vi "Main - On Load.vi"(8 "error in (no error)":errorcluster, 11 "Device Item Ref in":T1 format="%.0x") -> (0 "error out":errorcluster, 3 "Device Item Ref out":T1 format="%.0x")   [LabVIEW 2026, in "SEECD System Explorer.lvlib"]
uses:
  SEECD System Explorer.lvlib
  <vilib>/NI VeriStand/Custom Device API/Custom Device API.lvlib
  <vilib>/NI VeriStand/Custom Device API/Custom Device Channel Type.ctl
  <vilib>/NI VeriStand/Custom Device API/Custom Device Channel.ctl
  <vilib>/NI VeriStand/Custom Device Tools/Custom Device Utility Library/Custom Device Utility Library.lvlib
  Shared/Globals/Scan Engine GUIDs.vi
  Shared/SEECD Shared.lvlib
  Shared/Globals/Property Strings.vi
  <vilib>/NI VeriStand/Custom Device Tools/Custom Device Utility Library/NI VeriStand - Search for All Items by GUID.vi
  Shared/Globals/String Constants.vi
  <vilib>/NI VeriStand/Custom Device API/Set Item Property (Boolean).vi
  <vilib>/NI VeriStand/Custom Device API/Get Item Property (U32).vi
  <vilib>/NI VeriStand/Custom Device API/Set Item Property (String).vi
  C:/Users/Administrator/Desktop/Jatin/All DNC DLLs/NationalInstruments.VeriStand.SystemDefinitionAPI.dll
  Jatin/All DNC DLLs/NationalInstruments.VeriStand.SystemDefinitionAPI.dll
  <vilib>/NI VeriStand/Custom Device API/Custom Device Item Ref.ctl
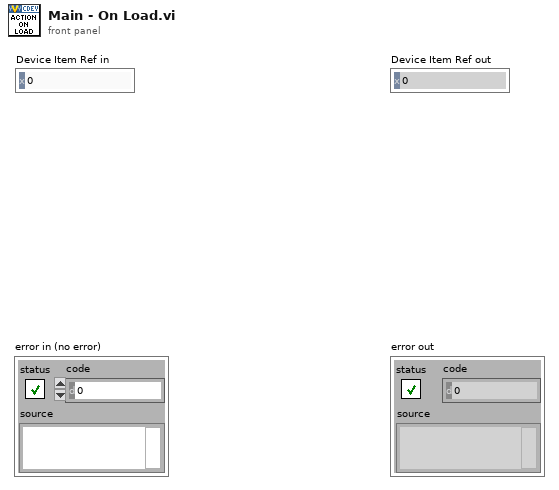
[diagram p1: front panel]
types:
  T1 = typedef "Custom Device API.lvlib/Custom Device Item Ref.ctl" = u64
  T2 = typedef "Custom Device API.lvlib/Custom Device Channel.ctl" = cluster{"Type":T3, "Units":string, "Default Value":dbl, "Faultable":bool, "Scalable":bool}
  T3 = typedef "Custom Device API.lvlib/Custom Device Channel Type.ctl" = enum16{"Input", "Output"}
  T4 = cluster{"Property Name Format String":string, "Offset":i32}
  T5 = typedef "Modules.lvlibp/Custom Device API.lvlib/Custom Device Item Ref.ctl" = u64
  T6 = typedef "Modules.lvlibp/RSI Module.lvclass/Module Models.ctl" = enum16{"Empty", "NI 9201", "NI 9203", "NI 9205", "NI 9206", "NI 9207", "NI 9208", "NI 9209", "NI 9210", "NI 9211", "NI 9212", "NI 9213", "NI 9214", "NI 9215", "NI 9216", "NI 9217", "NI 9219", "NI 9220", "NI 9221", "NI 9222", "NI 9223", "NI 9224", "NI 9225", "NI 9226", "NI 9227", "NI 9228", "NI 9229", "NI 9233", "NI 9234", "NI 9235", "NI 9236", "NI 9237", "NI 9239", "NI 9242", "NI 9244", "NI 9253", "NI 9263", "NI 9264", "NI 9265", "NI 9266", "NI 9269", "NI 9344", "NI 9350", "NI 9375", "NI 9401", "NI 9402", "NI 9403", "NI 9411", "NI 9421", "NI 9422", "NI 9423", "NI 9425", "NI 9426", "NI 9435", "NI 9436", "NI 9437", "NI 9472", "NI 9474", "NI 9475", "NI 9476", "NI 9477", "NI 9478", "NI 9481", "NI 9482", "NI 9485"}
  T7 = typedef "Modules.lvlibp/RSI Module.lvclass/Slot Settings.ctl" = cluster{"Slot":u32, "EtherCAT?":bool}
  T8 = typedef "Custom Device API.lvlib/Custom Device Item Info.ctl" = cluster{"Name":string, "Is Channel":bool, "GUID":string, "Is Waveform":bool}
  T9 = typedef "Custom Device API.lvlib/Custom Device File Dependency.ctl" = cluster{"Source":T10, "RT Destination":path, "ForceDownload?":bool, "SupportedTarget":T12, "Version":string}
  T10 = typedef "Custom Device API.lvlib/Path Specification.ctl" = cluster{"Path":path, "Type":T11}
  T11 = typedef "Custom Device API.lvlib/Path Type.ctl" = enum16{"Absolute", "To Base", "To Common Data Dir", "To Application Data Dir"}
  T12 = typedef "Custom Device API.lvlib/Custom Device Supported Target.ctl" = enum16{"All", "PharLap", "VxWorks", "Windows", "Linux_32_ARM", "Linux_x64", "PharLap & Windows", "PharLap & VxWorks", "VxWorks & Windows"}
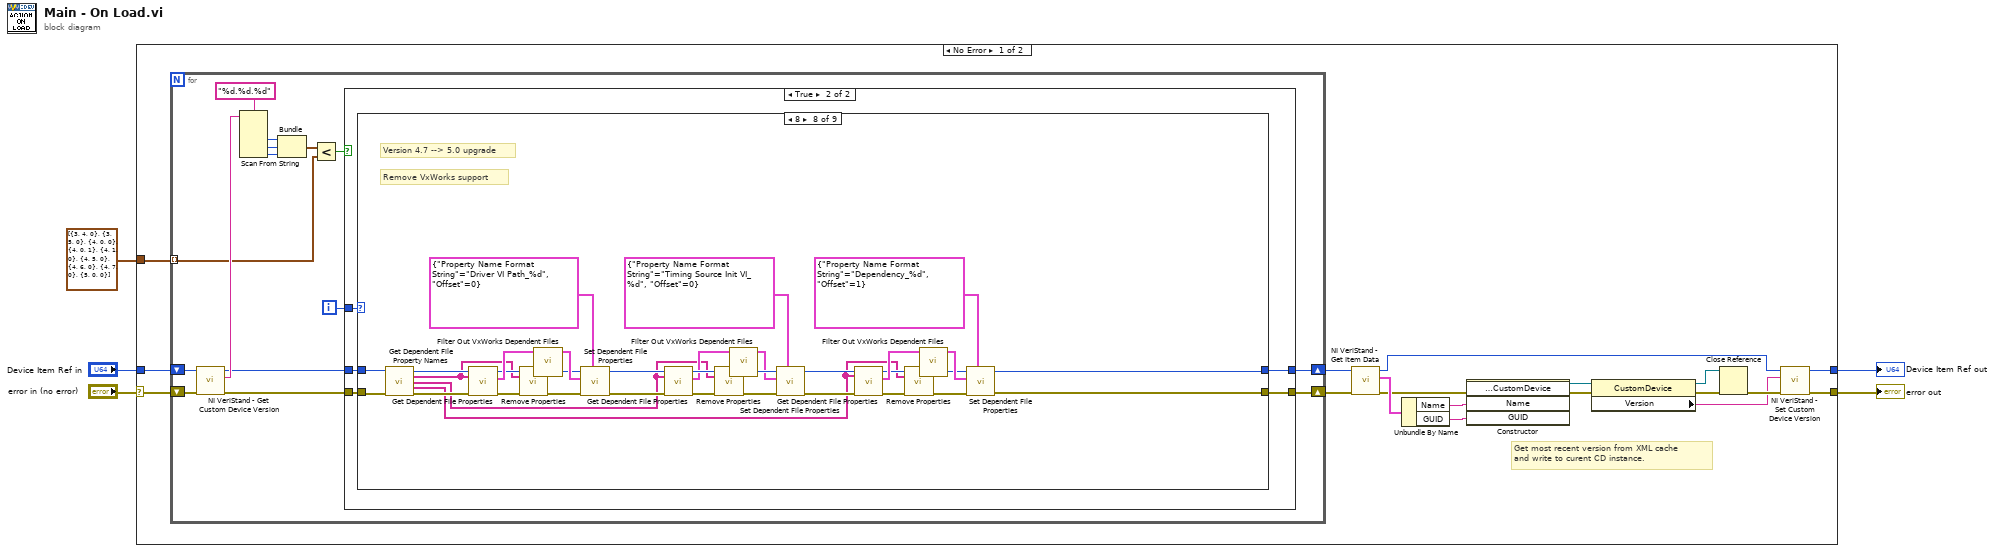
[diagram p0: block diagram]
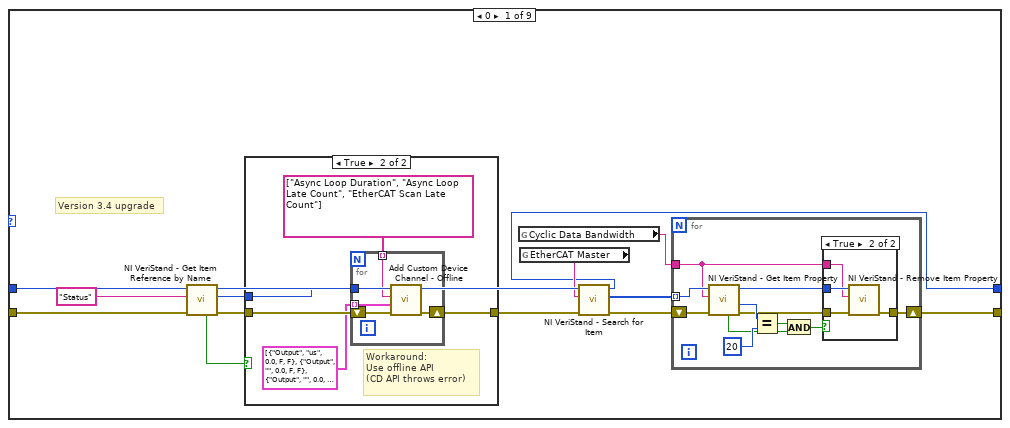
[diagram p3: hidden frame]
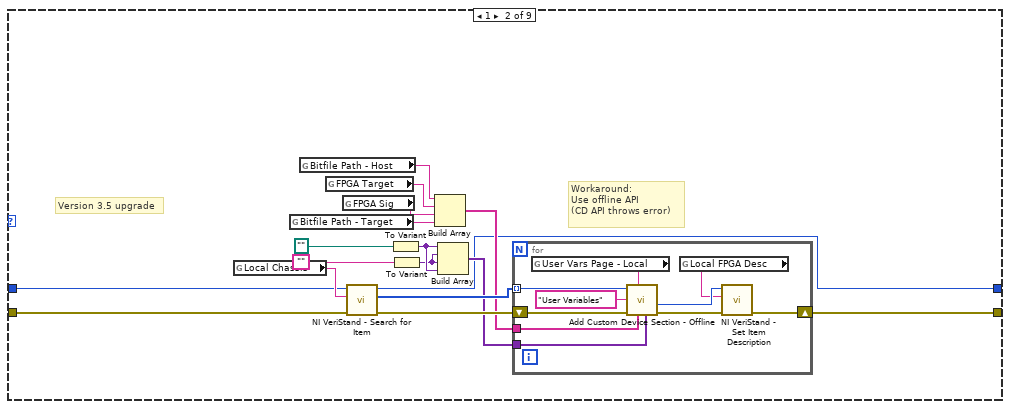
[diagram p6: hidden frame]
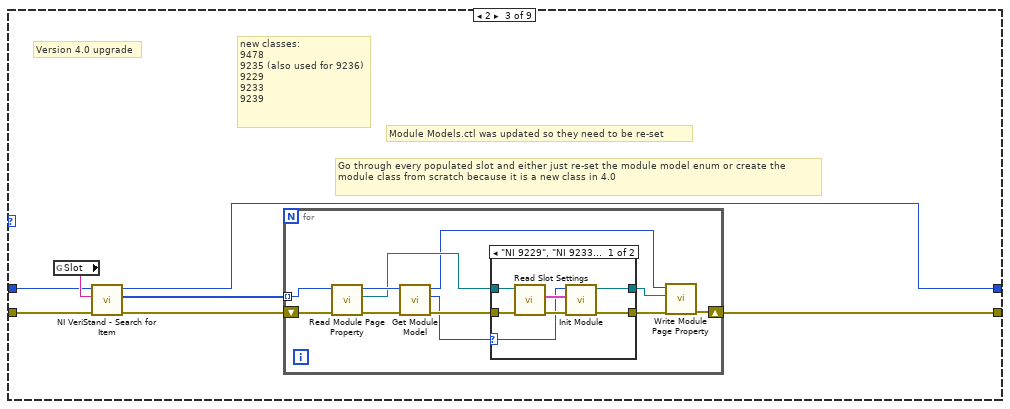
[diagram p7: hidden frame]
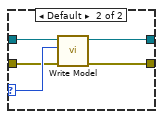
[diagram p8: hidden frame]
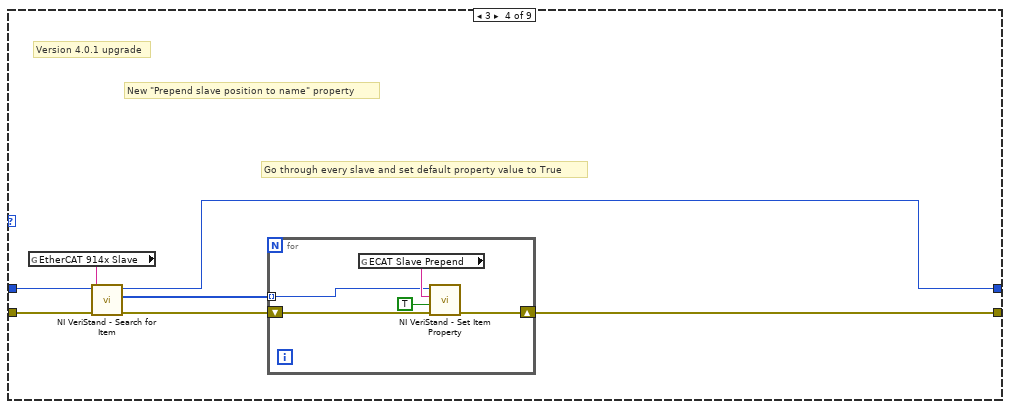
[diagram p9: hidden frame]
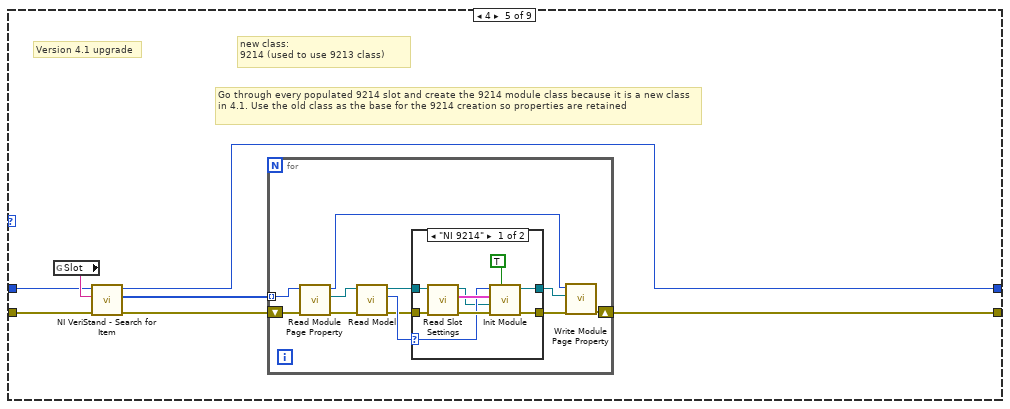
[diagram p10: hidden frame]
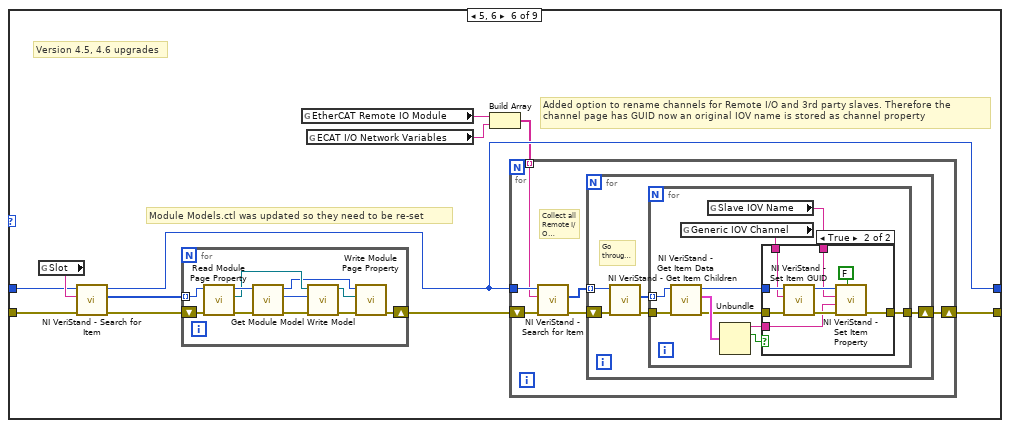
[diagram p12: hidden frame]
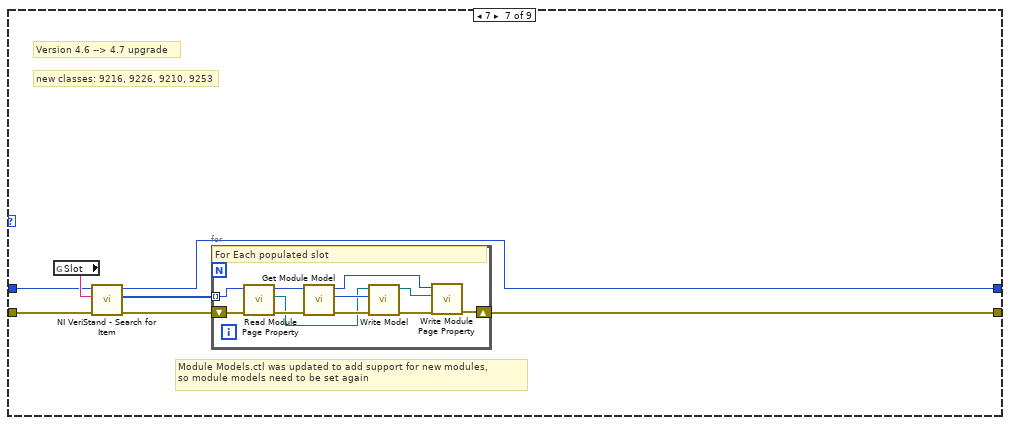
[diagram p14: hidden frame]
diagram:
  n1 = case shown="No Error" "error in (no error)" {
    selector: "error in (no error)" -> [w23 w293]
    tunnel: [w6 w293] -> w3
    tunnel: "Device Item Ref in" -> [w22 w292]
    tunnel: [w7 w292] -> w2
    tunnel: cluster{i32, i32, i32}[] [{3, 4, 0}, {3, 5, 0}, {4, 0, 0}, {4, 0, 1}, {4, 1, 0}, {4, 5, 0}, {4, 6, 0}, {4, 7, 0}, {5, 0, 0}] -> [w21 _]
    frame No Error {
      # "Get most recent version from XML cache\nand write to curent CD instance."
      n2 = for {
        shift-right: [w29] -> w19
        shift-left: w23 -> [w34]
        shift-right: [w27] -> w20
        shift-left: w22 -> [w33]
        tunnel: w21 -> [w24] mode=indexing
        i -> [w26]
        n3 = call <vilib>:"NI VeriStand - Get Custom Device Version.vi"("error in (no error)"=w34, "Device Ref in"=w33) -> ("error out"=w30:errorcluster, "Value"=w32:string, "Device Ref out"=w28:T1)  [unwired: 7 in]
        n4 = Scan From String(format string="%d.%d.%d", input string=w32) -> (output 1=w36:i32, output 2=w37:i32, output 3=w25:i32)  [unwired: 5 in, 3 out]
        n5 = Bundle(w36, w37, w25) -> (w38:cluster{i32, i32, i32})  [unwired: 1 in]
        n6 = Less?(x=w38, y=w24) -> (x < y?=w31:bool)
        n7 = case shown="True" w31 {
          tunnel: w30 -> [w40 w45]
          tunnel: [w40 w44] -> w29
          tunnel: w28 -> [w39 w41]
          tunnel: [w39 w42] -> w27
          tunnel: w26 -> [_ w43]
          frame False {
          }
          frame True {
            n8 = case shown="8" w43 {
              tunnel: w45 -> [w46 w89 w116 w146 w158 w191 w240 w278 w291]
              tunnel: [w52 w88 w115 w145 w157 w190 w239 w262 w291] -> w44
              tunnel: [w54 w87 w114 w144 w156 w188 w238 w263 w290] -> w42
              tunnel: w41 -> [w47 w90 w117 w147 w159 w192 w241 w289 w290]
              frame 0 {
                # "Version 3.4 upgrade"
                n9 = call <vilib>:"NI VeriStand - Get Item Reference by Name.vi"("error in (no error)"=w46, "Item Name"="Status" ("Section Name"), "Parent Ref in"=w47) -> ("error out"=w50:errorcluster, "Item Ref"=w49:T1, "Parent Ref out"=w58:T1, "Found"=w48:bool)  [unwired: 5 in]
                n10 = case shown="True" w48 {
                  tunnel: w49 -> [_ w65]
                  tunnel: w50 -> [w60 w64]
                  tunnel: [w60 w63] -> w59
                  frame False {
                  }
                  frame True {
                    # "Workaround:\nUse offline API\n(CD API throws error)"
                    n11 = for {
                      tunnel: w65 -> [w68]
                      shift-right: [w70] -> w63
                      shift-left: w64 -> [w69]
                      tunnel: T2[] [{"Type"=enum."Output", "Units"="us", "Default Value"=0.0, "Faultable"=FALSE, "Scalable"=FALSE}, {"Type"=enum."Output", "Units"="", "Default Value"=0.0, "Faultable"=FALSE, "Scalable"=FALSE}, {"Type"=enum."Output", "Units"="", "Default Value"=0.0, "Faultable"=FALSE, "Scalable"=FALSE}] -> [w66] mode=indexing
                      tunnel: string[] ["Async Loop Duration", "Async Loop Late Count", "EtherCAT Scan Late Count"] -> [w67] mode=indexing
                      n12 = call "Add Custom Device Channel - Offline.vi"("error in (no error)"=w69, "Channel"=w66, "Channel Name"=w67, "Parent Ref in"=w68) -> ("error out"=w70:errorcluster)  [unwired: 4 in, 3 out]
                    }
                  }
                }
                n13 = global read "Property Strings.vi" "Cyclic Data Bandwidth"() -> (w53:string)
                n14 = global read "Scan Engine GUIDs.vi" "EtherCAT Master"() -> (w57:string)
                n15 = call-poly <vilib>:"NI VeriStand - Search for Item.vi"("error in"=w59, "Item GUID"=w57, "Section Ref in"=w58) -> ("error out"=w55:errorcluster, "Item Refs"=w56:T1[], "Section Ref out"=w54:T1)  [unwired: 5 in, 1 out]
                n16 = for {
                  tunnel: w56 -> [w80] mode=indexing
                  shift-right: [w71] -> w52
                  shift-left: w55 -> [w81]
                  tunnel: w53 -> [w72]
                  n17 = call-poly <vilib>:"NI VeriStand - Get Item Property.vi"("error in (no error)"=w81, "Property Name"=w72, "Item Ref in"=w80) -> ("error out"=w74:errorcluster, "Value"=w79:u32, "Item Ref out"=w73:T1, "Found?"=w76:bool)  [unwired: 5 in]
                  n18 = Equal?(x=w79, y=u32 20 ("x")) -> (x = y?=w77:bool)
                  n19 = And(x=w77, y=w76) -> (x .and. y?=w75:bool)
                  n20 = case shown="True" w75 {
                    tunnel: w74 -> [w82 w85]
                    tunnel: w73 -> [_ w86]
                    tunnel: w72 -> [_ w84]
                    tunnel: [w82 w83] -> w71
                    frame False {
                    }
                    frame True {
                      n21 = call <vilib>:"NI VeriStand - Remove Item Property.vi"("error in (no error)"=w85, "Property Name"=w84, "Item Ref in"=w86) -> ("error out"=w83:errorcluster)  [unwired: 6 in, 2 out]
                    }
                  }
                }
              }
              frame 1 {
                # "Workaround:\nUse offline API\n(CD API throws error)"
                # "Version 3.5 upgrade"
                n22 = global read "Scan Engine GUIDs.vi" "Local Chassis"() -> (w101:string)
                n23 = global read "Property Strings.vi" "Bitfile Path - Target"() -> (w94:string)
                n24 = global read "Property Strings.vi" "Bitfile Path - Host"() -> (w97:string)
                n25 = global read "Property Strings.vi" "FPGA Target"() -> (w96:string)
                n26 = global read "Property Strings.vi" "FPGA Sig"() -> (w95:string)
                n27 = call-poly <vilib>:"NI VeriStand - Search for Item.vi"("error in"=w89, "Item GUID"=w101, "Section Ref in"=w90) -> ("error out"=w103:errorcluster, "Item Refs"=w102:T1[], "Section Ref out"=w87:T1)  [unwired: 5 in, 1 out]
                n28 = To Variant(anything=path "") -> (Variant=w93:variant)
                n29 = To Variant(anything="") -> (Variant=w91:variant)
                n30 = Build Array(w97, w96, w95, w94) -> (w99:string[])
                n31 = Build Array(w93, w91, w91, w93) -> (w100:variant[])
                n32 = for {
                  tunnel: w99 -> [w112]
                  tunnel: w100 -> [w111]
                  shift-right: [w106] -> w88
                  shift-left: w103 -> [w113]
                  tunnel: w102 -> [w110] mode=indexing
                  n33 = global read "Scan Engine GUIDs.vi" "User Vars Page - Local"() -> (w109:string)
                  n34 = call "Add Custom Device Section - Offline.vi"("Property Values"=w111, "Property names"=w112, "GUID (Default Section)"=w109, "error in (no error)"=w113, "Section Name"="User Variables", "Parent Ref in"=w110) -> ("error out"=w107:errorcluster, "Section Ptr"=w105:T1)  [unwired: 2 in, 2 out]
                  n35 = global read "String Constants.vi" "Local FPGA Desc"() -> (w104:string)
                  n36 = call <vilib>:"NI VeriStand - Set Item Description.vi"("error in (no error)"=w107, "Description"=w104, "Item Ref in"=w105) -> ("error out"=w106:errorcluster)  [unwired: 6 in, 2 out]
                }
              }
              frame 2 {
                # "new classes:\n9478\n9235 (also used for 9236)\n9229\n9233\n9239"
                # "Go through every populated slot and either just re-set the module model enum or create the module class from scratch because it is a new class in 4.0"
                # "Module Models.ctl was updated so they need to be re-set"
                # "Version 4.0 upgrade"
                n37 = global read "Scan Engine GUIDs.vi" "Slot"() -> (w118:string)
                n38 = call-poly <vilib>:"NI VeriStand - Search for Item.vi"("error in"=w116, "Item GUID"=w118, "Section Ref in"=w117) -> ("error out"=w120:errorcluster, "Item Refs"=w119:T1[], "Section Ref out"=w114:T1)  [unwired: 5 in, 1 out]
                n39 = for {
                  shift-right: [w131] -> w115
                  shift-left: w120 -> [w127]
                  tunnel: w119 -> [w128] mode=indexing
                  n40 = call "Read Module Page Property.vi"("error in (no error)"=w127, "Node Ptr In"=w128) -> ("error out"=w130:errorcluster, "RSI Module"=w125:refnum<class "RSI Module.lvclass">, "Node Ptr Out"=w129:T5)  [unwired: 7 in]
                  n41 = call "Get Module Model.vi"("error in (no error)"=w130, "Item Ref in"=w129) -> ("error out"=w122:errorcluster, "Module"=w121:T6, "Item Ref out"=w123:T1)  [unwired: 7 in]
                  n42 = case shown="\"NI 9229\", \"NI 9233\", \"NI 9235\", \"NI 9236\", \"NI 9239\", \"NI 9478\"" w121 {
                    selector: w121 -> [w135 w142]
                    tunnel: [w134 w143] -> w126
                    tunnel: w125 -> [w136 w141]
                    tunnel: [w133 w140] -> w124
                    tunnel: w122 -> [w132 w139]
                    frame "NI 9229", "NI 9233", "NI 9235", "NI 9236", "NI 9239", "NI 9478" {
                      n43 = call "Read Slot Settings.vi"("error in (no error)"=w132, "RSI Module in"=w136) -> ("error out"=w137:errorcluster, "Slot Settings"=w138:T7)  [unwired: 7 in, 1 out]
                      n44 = call "Init Module.vi"("error in (no error)"=w137, "Slot Settings"=w138, "Module Model"=w135) -> ("error out"=w134:errorcluster, "RSI Module out"=w133:refnum<class "RSI Module.lvclass">)  [unwired: 7 in]
                    }
                    frame Default {
                      n45 = call "Write Model.vi"("error in (no error)"=w139, "Model"=w142, "RSI Module in"=w141) -> ("error out"=w143:errorcluster, "RSI Module out"=w140:refnum<class "RSI Module.lvclass">)  [unwired: 7 in]
                    }
                  }
                  n46 = call "Write Module Page Property.vi"("error in (no error)"=w126, "RSI Module"=w124, "Node Ptr In"=w123) -> ("error out"=w131:errorcluster)  [unwired: 6 in, 2 out]
                }
              }
              frame 3 {
                # "New \"Prepend slave position to name\" property"
                # "Go through every slave and set default property value to True"
                # "Version 4.0.1 upgrade"
                n47 = global read "Scan Engine GUIDs.vi" "EtherCAT 914x Slave"() -> (w148:string)
                n48 = call-poly <vilib>:"NI VeriStand - Search for Item.vi"("error in"=w146, "Item GUID"=w148, "Section Ref in"=w147) -> ("error out"=w150:errorcluster, "Item Refs"=w149:T1[], "Section Ref out"=w144:T1)  [unwired: 5 in, 1 out]
                n49 = for {
                  shift-right: [w151] -> w145
                  shift-left: w150 -> [w155]
                  tunnel: w149 -> [w153] mode=indexing
                  n50 = global read "Property Strings.vi" "ECAT Slave Prepend"() -> (w154:string)
                  n51 = call-poly <vilib>:"NI VeriStand - Set Item Property.vi"("error in (no error)"=w155, "Value"=TRUE, "Property Name"=w154, "Item Ref in"=w153) -> ("error out"=w151:errorcluster)  [unwired: 5 in, 2 out]
                }
              }
              frame 4 {
                # "new class:\n9214 (used to use 9213 class)"
                # "Go through every populated 9214 slot and create the 9214 module class because it is a new class in 4.1. Use the old class as the base for the 9214 creation so properties are retained"
                # "Version 4.1 upgrade"
                n52 = global read "Scan Engine GUIDs.vi" "Slot"() -> (w160:string)
                n53 = call-poly <vilib>:"NI VeriStand - Search for Item.vi"("error in"=w158, "Item GUID"=w160, "Section Ref in"=w159) -> ("error out"=w162:errorcluster, "Item Refs"=w161:T1[], "Section Ref out"=w156:T1)  [unwired: 5 in, 1 out]
                n54 = for {
                  shift-right: [w173] -> w157
                  shift-left: w162 -> [w171]
                  tunnel: w161 -> [w172] mode=indexing
                  n55 = call "Read Module Page Property.vi"("error in (no error)"=w171, "Node Ptr In"=w172) -> ("error out"=w168:errorcluster, "RSI Module"=w167:refnum<class "RSI Module.lvclass">, "Node Ptr Out"=w163:T5)  [unwired: 7 in]
                  n56 = call "Read Model.vi"("error in (no error)"=w168, "RSI Module in"=w167) -> ("error out"=w164:errorcluster, "Model"=w165:T6, "RSI Module out"=w166:refnum<class "RSI Module.lvclass">)  [unwired: 7 in]
                  n57 = case shown="\"NI 9214\"" w165 {
                    selector: w165 -> [w180 _]
                    tunnel: w164 -> [w179 w184]
                    tunnel: [w175 w184] -> w170
                    tunnel: w166 -> [w176 w183]
                    tunnel: [w174 w183] -> w169
                    frame "NI 9214" {
                      n58 = call "Read Slot Settings.vi"("error in (no error)"=w179, "RSI Module in"=w176) -> ("error out"=w181:errorcluster, "Slot Settings"=w182:T7, "RSI Module out"=w177:refnum<class "RSI Module.lvclass">)  [unwired: 7 in]
                      n59 = call "Init Module.vi"("Create from class input? (F)"=TRUE, "error in (no error)"=w181, "RSI Module in"=w177, "Slot Settings"=w182, "Module Model"=w180) -> ("error out"=w175:errorcluster, "RSI Module out"=w174:refnum<class "RSI Module.lvclass">)  [unwired: 5 in]
                    }
                    frame Default {
                    }
                  }
                  n60 = call "Write Module Page Property.vi"("error in (no error)"=w170, "RSI Module"=w169, "Node Ptr In"=w163) -> ("error out"=w173:errorcluster)  [unwired: 6 in, 2 out]
                }
              }
              frame 5, 6 {
                # "Added option to rename channels for Remote I/O and 3rd party slaves. Therefore the\nchannel page has GUID now an original IOV name is stored as channel property"
                # "Module Models.ctl was updated so they need to be re-set"
                # "Version 4.5, 4.6 upgrades"
                n61 = global read "Scan Engine GUIDs.vi" "Slot"() -> (w193:string)
                n62 = call-poly <vilib>:"NI VeriStand - Search for Item.vi"("error in"=w191, "Item GUID"=w193, "Section Ref in"=w192) -> ("error out"=w195:errorcluster, "Item Refs"=w194:T1[], "Section Ref out"=w188:T1)  [unwired: 5 in, 1 out]
                n63 = for {
                  shift-right: [w237] -> w189
                  shift-left: w195 -> [w233]
                  tunnel: w194 -> [w234] mode=indexing
                  n64 = call "Read Module Page Property.vi"("error in (no error)"=w233, "Node Ptr In"=w234) -> ("error out"=w236:errorcluster, "RSI Module"=w229:refnum<class "RSI Module.lvclass">, "Node Ptr Out"=w235:T5)  [unwired: 7 in]
                  n65 = call "Get Module Model.vi"("error in (no error)"=w236, "Item Ref in"=w235) -> ("error out"=w232:errorcluster, "Module"=w231:T6, "Item Ref out"=w227:T1)  [unwired: 7 in]
                  n66 = call "Write Model.vi"("error in (no error)"=w232, "Model"=w231, "RSI Module in"=w229) -> ("error out"=w230:errorcluster, "RSI Module out"=w228:refnum<class "RSI Module.lvclass">)  [unwired: 7 in]
                  n67 = call "Write Module Page Property.vi"("error in (no error)"=w230, "RSI Module"=w228, "Node Ptr In"=w227) -> ("error out"=w237:errorcluster)  [unwired: 6 in, 2 out]
                }
                n68 = global read "Scan Engine GUIDs.vi" "EtherCAT Remote IO Module"() -> (w187:string)
                n69 = global read "Scan Engine GUIDs.vi" "ECAT I/O Network Variables"() -> (w186:string)
                n70 = Build Array(w187, w186) -> (w185:string[])
                n71 = for {
                  tunnel: w188 -> [w200]
                  tunnel: w185 -> [w199] mode=indexing
                  shift-right: [w198] -> w190
                  shift-left: w189 -> [w201]
                  # "Collect all Remote I/O modules and all I/O sections of all 3rd party slaves"
                  n72 = call-poly <vilib>:"NI VeriStand - Search for Item.vi"("error in"=w201, "Item GUID"=w199, "Section Ref in"=w200) -> ("error out"=w197:errorcluster, "Item Refs"=w196:T1[])  [unwired: 5 in, 2 out]
                  n73 = for {
                    shift-right: [w204] -> w198
                    shift-left: w197 -> [w205]
                    tunnel: w196 -> [w206] mode=indexing
                    # "Go through every I/O in all sections to change it's page GUID for default to \"Generic IOV Channel\" and copy channel name to the new property \"Slave IOV Name\" to be used in later on in the RT Driver VI. As user can change channel name this property stores IOV name/path returned by the EtherCAT driver"
                    n74 = call <vilib>:"NI VeriStand - Get Item Children.vi"("error in (no error)"=w205, "Item Ref in"=w206) -> ("error out"=w203:errorcluster, "Child Refs"=w202:T1[])  [unwired: 6 in, 2 out]
                    n75 = for {
                      tunnel: [w212] -> w204
                      tunnel: w203 -> [w215]
                      tunnel: w202 -> [w214] mode=indexing
                      n76 = call <vilib>:"NI VeriStand - Get Item Data.vi"("error in (no error)"=w215, "Item Ref in"=w214) -> ("error out"=w209:errorcluster, "Item Info"=w216:T8, "Item Ref out"=w210:T1)  [unwired: 6 in, 1 out]
                      n77 = global read "Scan Engine GUIDs.vi" "Generic IOV Channel"() -> (w208:string)
                      n78 = global read "Property Strings.vi" "Slave IOV Name"() -> (w207:string)
                      n79 = Unbundle(w216) -> ("Name"=w213:string, "Is Channel"=w211:bool)  [unwired: 2 out]
                      n80 = case shown="True" w211 {
                        tunnel: [w217 w222] -> w212
                        tunnel: w210 -> [_ w226]
                        tunnel: w209 -> [w217 w225]
                        tunnel: w208 -> [_ w220]
                        tunnel: w207 -> [_ w219]
                        tunnel: w213 -> [_ w218]
                        frame False {
                        }
                        frame True {
                          n81 = call <vilib>:"NI VeriStand - Set Item GUID.vi"("error in (no error)"=w225, "GUID"=w220, "Item Ref in"=w226) -> ("error out"=w223:errorcluster, "Item Ref out"=w224:T1)  [unwired: 7 in]
                          n82 = call-poly <vilib>:"NI VeriStand - Set Item Property.vi"("Binary String (T)"=FALSE, "error in (no error)"=w223, "Value"=w218, "Property Name"=w219, "Item Ref in"=w224) -> ("error out"=w222:errorcluster)  [unwired: 4 in, 2 out]
                        }
                      }
                    }
                  }
                }
              }
              frame 7 {
                # "new classes: 9216, 9226, 9210, 9253"
                # "Module Models.ctl was updated to add support for new modules, \nso module models need to be set again"
                # "Version 4.6 --> 4.7 upgrade"
                n83 = global read "Scan Engine GUIDs.vi" "Slot"() -> (w242:string)
                n84 = call-poly <vilib>:"NI VeriStand - Search for Item.vi"("error in"=w240, "Item GUID"=w242, "Section Ref in"=w241) -> ("error out"=w244:errorcluster, "Item Refs"=w243:T1[], "Section Ref out"=w238:T1)  [unwired: 5 in, 1 out]
                n85 = for {
                  shift-right: [w255] -> w239
                  shift-left: w244 -> [w251]
                  tunnel: w243 -> [w252] mode=indexing
                  # "For Each populated slot"
                  n86 = call "Read Module Page Property.vi"("error in (no error)"=w251, "Node Ptr In"=w252) -> ("error out"=w254:errorcluster, "RSI Module"=w245:refnum<class "RSI Module.lvclass">, "Node Ptr Out"=w253:T5)  [unwired: 7 in]
                  n87 = call "Get Module Model.vi"("error in (no error)"=w254, "Item Ref in"=w253) -> ("error out"=w247:errorcluster, "Module"=w246:T6, "Item Ref out"=w248:T1)  [unwired: 7 in]
                  n88 = call "Write Model.vi"("error in (no error)"=w247, "Model"=w246, "RSI Module in"=w245) -> ("error out"=w250:errorcluster, "RSI Module out"=w249:refnum<class "RSI Module.lvclass">)  [unwired: 7 in]
                  n89 = call "Write Module Page Property.vi"("error in (no error)"=w250, "RSI Module"=w249, "Node Ptr In"=w248) -> ("error out"=w255:errorcluster)  [unwired: 6 in, 2 out]
                }
              }
              frame 8 {
                # "Remove VxWorks support"
                # "Version 4.7 --> 5.0 upgrade"
                n90 = call "Get Dependent File Property Names.vi"("Device Ref in"=w289, "error in (no error)"=w278) -> ("Device Ref out"=w288:T1, "driver vi path properties"=w280:string[], "timing source properties"=w259:string[], "dependency properties"=w258:string[], "error out"=w287:errorcluster)  [unwired: 9 in]
                n91 = call "Get Dependent File Properties.vi"("error in (no error)"=w287, "property names"=w280, "Device Ref in"=w288) -> ("error out"=w282:errorcluster, "property values"=w286:T9[], "Device Ref out"=w284:T1)  [unwired: 6 in]
                n92 = call "Remove Properties.vi"("error in (no error)"=w282, "property names"=w280, "Device Ref in"=w284) -> ("error out"=w281:errorcluster, "Device Ref out"=w283:T1)  [unwired: 7 in]
                n93 = call "Filter Out VxWorks Dependent Files.vi"("dependent files in"=w286) -> ("dependent files out"=w285:T9[])  [unwired: 10 in]
                n94 = call "Set Dependent File Properties.vi"("Format Settings"=T4 {"Property Name Format String"="Driver VI Path_%d", "Offset"=0}, "error in (no error)"=w281, "Dependent Files"=w285, "Device Ref in"=w283) -> ("error out"=w260:errorcluster, "Device Ref out"=w265:T1)  [unwired: 6 in]
                n95 = call "Get Dependent File Properties.vi"("error in (no error)"=w260, "property names"=w259, "Device Ref in"=w265) -> ("error out"=w276:errorcluster, "property values"=w272:T9[], "Device Ref out"=w274:T1)  [unwired: 6 in]
                n96 = call "Remove Properties.vi"("error in (no error)"=w276, "property names"=w259, "Device Ref in"=w274) -> ("error out"=w277:errorcluster, "Device Ref out"=w275:T1)  [unwired: 7 in]
                n97 = call "Filter Out VxWorks Dependent Files.vi"("dependent files in"=w272) -> ("dependent files out"=w273:T9[])  [unwired: 10 in]
                n98 = call "Set Dependent File Properties.vi"("Format Settings"=T4 {"Property Name Format String"="Timing Source Init VI_%d", "Offset"=0}, "error in (no error)"=w277, "Dependent Files"=w273, "Device Ref in"=w275) -> ("error out"=w261:errorcluster, "Device Ref out"=w264:T1)  [unwired: 6 in]
                n99 = call "Get Dependent File Properties.vi"("error in (no error)"=w261, "property names"=w258, "Device Ref in"=w264) -> ("error out"=w267:errorcluster, "property values"=w271:T9[], "Device Ref out"=w269:T1)  [unwired: 6 in]
                n100 = call "Remove Properties.vi"("error in (no error)"=w267, "property names"=w258, "Device Ref in"=w269) -> ("error out"=w266:errorcluster, "Device Ref out"=w268:T1)  [unwired: 7 in]
                n101 = call "Filter Out VxWorks Dependent Files.vi"("dependent files in"=w271) -> ("dependent files out"=w270:T9[])  [unwired: 10 in]
                n102 = call "Set Dependent File Properties.vi"("Format Settings"=T4 {"Property Name Format String"="Dependency_%d", "Offset"=1}, "error in (no error)"=w266, "Dependent Files"=w270, "Device Ref in"=w268) -> ("error out"=w262:errorcluster, "Device Ref out"=w263:T1)  [unwired: 6 in]
              }
              frame Default {
              }
            }
          }
        }
      }
      n103 = call <vilib>:"NI VeriStand - Get Item Data.vi"("error in (no error)"=w19, "Item Ref in"=w20) -> ("error out"=w15:errorcluster, "Item Info"=w18:T8, "Item Ref out"=w8:T1)  [unwired: 6 in, 1 out]
      n104 = Unbundle By Name(w18) -> ("Name"=w17:string, "GUID"=w16:string)
      n105 = constructor class="CustomDevice"(error in=w15, "Name"=w17, "GUID"=w16) -> (reference out=w14:refnum<k39>, error out=w13:errorcluster)  [unwired: 2 in, 3 out]
      n106 = property class="CustomDevice"(reference=w14, error in=w13) -> (reference out=w11:refnum<k39>, error out=w12:errorcluster, "Version"=w9:string)
      n107 = Close Reference(reference=w11, error in (no error)=w12) -> (error out=w10:errorcluster)
      n108 = call <vilib>:"NI VeriStand - Set Custom Device Version.vi"("error in (no error)"=w10, "Value"=w9, "Device Ref in"=w8) -> ("error out"=w6:errorcluster, "Device Ref out"=w7:T1)  [unwired: 7 in]
    }
    frame Error {
    }
  }
  "error out" <- w3
  "Device Item Ref out" <- w2
